vi "Logging_CloseLogfile.vi"(8 "error in (no error)":errorcluster, 11 "Byte Stream File in":refnum<file>) -> (0 "error out":errorcluster)   [LabVIEW 2014]
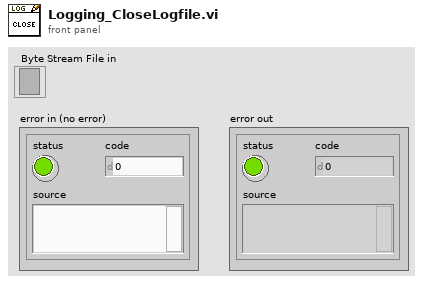
[diagram p1: front panel]
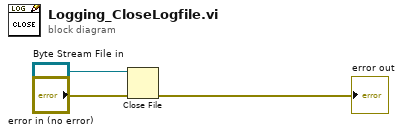
[diagram p0: block diagram]
diagram:
  n1 = Close File(refnum="Byte Stream File in", error in="error in (no error)") -> (error out=→"error out":errorcluster)  [unwired: 1 out]
